vi "Convert-Speaker to Tag.vi"(1 "Speaker":T1(ring)) -> (0 "Tag":string)   [LabVIEW 2015]
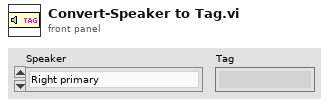
[diagram p1: front panel]
types:
  T1 = enum16{"Right primary", "Right secondary", "Left primary", "Left secondary"}
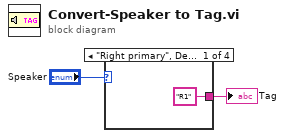
[diagram p0: block diagram]
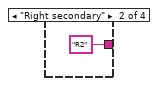
[diagram p2: hidden frame]
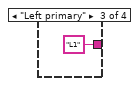
[diagram p3: hidden frame]
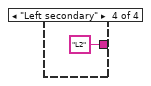
[diagram p4: hidden frame]
diagram:
  n1 = case shown="\"Right primary\", Default" "Speaker" {
    tunnel: ["R1" "R2" "L1" "L2"] -> w2
    frame "Right primary", Default {
    }
    frame "Right secondary" {
    }
    frame "Left primary" {
    }
    frame "Left secondary" {
    }
  }
  "Tag" <- w2
